vi "Handle Processing Error.vi"(8 "error in (no error)":errorcluster, 11 "StreamWriter in":refnum<class "Sift Stream.lvclass">) -> (0 "error out":errorcluster, 2 "Error Response":T1, 3 "StreamWriter out":refnum<class "Sift Stream.lvclass">)   [LabVIEW 2024, in "Sift Stream.lvlib" / "Sift Stream.lvclass"]
uses:
  Sift Stream.lvclass
  <vilib>/FlexLogger/SDK/PluginSDK.lvlibp/PEFClasses/SDK/Processing Element/Error Response Type.ctl
  Sift Stream.lvclass/Sift Stream.ctl
  <vilib>/FlexLogger/SDK/PluginSDK.lvlibp/PEFClasses/SDK/Processing Element/Processing Element.lvclass
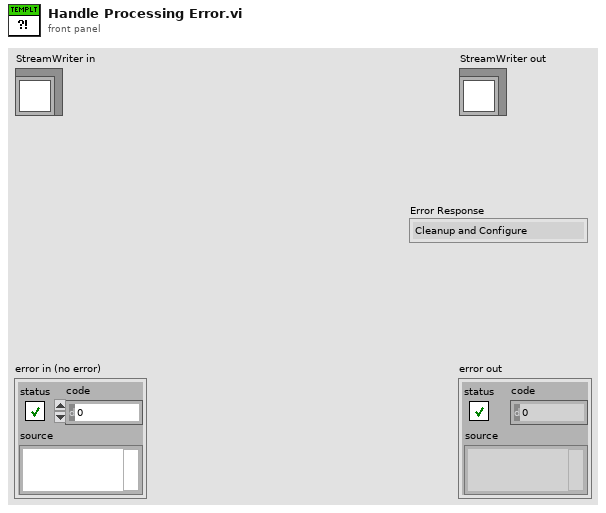
[diagram p1: front panel]
types:
  T1 = typedef "PluginSDK.lvlibp/Processing Element.lvclass/Error Response Type.ctl" = enum16{"Cleanup and Configure", "Cleanup and Finalize", "Report and Continue"}
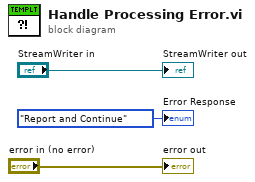
[diagram p0: block diagram]
diagram:
  "error out" <- "error in (no error)"
  "StreamWriter out" <- "StreamWriter in"
  "Error Response" <- Error_Response_Type."Report and Continue" ("Error Response")
